vi "Encode Internal Text.vi"(1 "string":string) -> (0 "data":u8[](array[numeric]))   [LabVIEW 2020, in "NI_SFTP.lvlib"]
uses:
  <vilib>/net/SFTP/NI_SFTP.lvlib
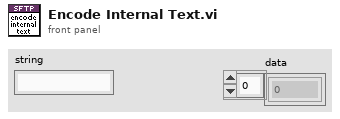
[diagram p1: front panel]
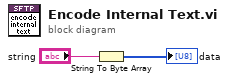
[diagram p0: block diagram]
diagram:
  n1 = String To Byte Array(string="string") -> (unsigned byte array=→"data":u8[])
